vi "testGetArrayNotAssignedValueIdx.vi"(8 "error in (no error)":errorcluster) -> (0 "error out":errorcluster)   [LabVIEW 2016]
doc: "Test to get the not-assigned-value index array."
uses:
  <vilib>/addons/_JKI Toolkits/Caraya/classes/Assert/Assert.lvclass
  <vilib>/addons/_JKI Toolkits/Caraya/classes/Test/Test.lvclass
  MatOper/MatOper.lvclass
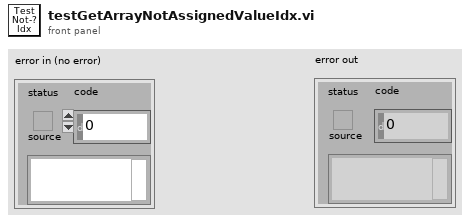
[diagram p1: front panel]
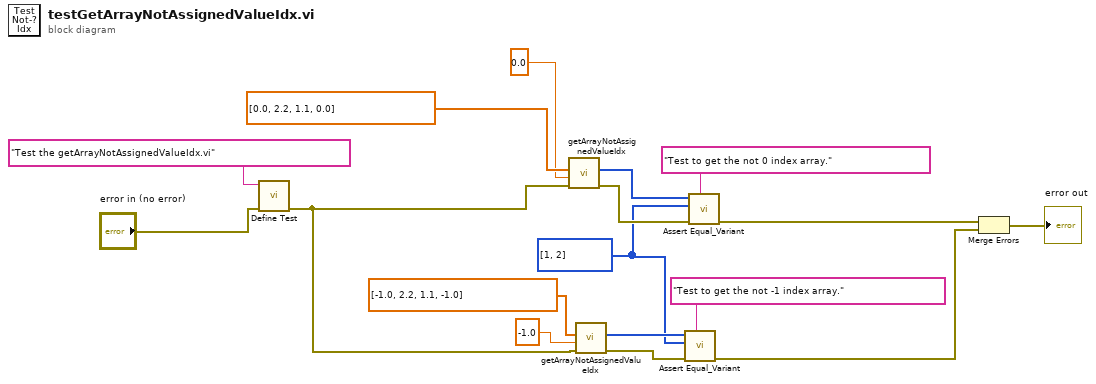
[diagram p0: block diagram]
diagram:
  w6 = i32[] [1, 2] ("Index Array")
  n1 = call <vilib>:"Define Test.vi"("error in (no error)"="error in (no error)", "Label (VI Title)"="Test the getArrayNotAssignedValueIdx.vi") -> ("error out"=w8:errorcluster)  [unwired: 9 in]
  n2 = call "getArrayNotAssignedValueIdx.vi"("error in (no error)"=w8, "Assigned Value"=0.0, "Array"=dbl[] [0.0, 2.2, 1.1, 0.0]) -> ("error out"=w15:errorcluster, "Index Array"=w14:i32[])  [unwired: 6 in, 1 out]
  n3 = call "getArrayNotAssignedValueIdx.vi"("error in (no error)"=w8, "Assigned Value"=-1.0, "Array"=dbl[] [-1.0, 2.2, 1.1, -1.0]) -> ("error out"=w5:errorcluster, "Index Array"=w7:i32[])  [unwired: 6 in, 1 out]
  n4 = call <vilib>:"Assert Equal_Variant.vi"("Label"="Test to get the not -1 index array.", "error in (no error)"=w5, "Y"=w6, "X"=w7) -> ("error out"=w2:errorcluster)  [unwired: 7 in]
  n5 = call <vilib>:"Assert Equal_Variant.vi"("Label"="Test to get the not 0 index array.", "error in (no error)"=w15, "Y"=w6, "X"=w14) -> ("error out"=w4:errorcluster)  [unwired: 7 in]
  n6 = Merge Errors(w4, w2) -> (→"error out":errorcluster)
